vi "Calculation chance.vi"(2 "Defective (%)":dbl) -> (0 "Defect":bool)   [LabVIEW 2020]
uses:
  <vilib>/express/express arith-compare/Formula/XNode/ExpressFormulaBlockNode.xnode
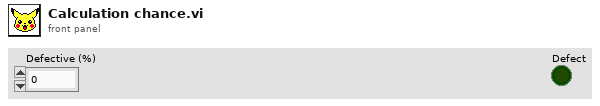
[diagram p1: front panel]
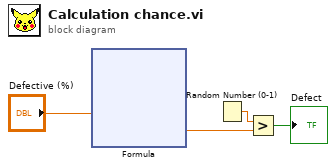
[diagram p0: block diagram]
diagram:
  n1 = xnode "Formula"("X1"="Defective (%)") -> ("Result"=w3:dbl)  [unwired: 1 in, 1 out]
  n2 = Random Number (0-1)() -> (number: 0 to 1=w2:dbl)
  n3 = Greater?(x=w2, y=w3) -> (0:→"Defect":bool)
